vi "4155C QSCV Config SMUs v2.0.vi"(0 "VISA resource name in":refnum<visa-resource-name>, 1 "QSCV - Probe 4":u32(ring)=3 items=["SMU1  ", "SMU2  ", "SMU3  ", "SMU4  ", "SMU5  ", "SMU6  "], 2 "Gate mode":u16(ring) items=["Auto", "Limited", "Fixed"], 3 "Gate Range":u8(slide)=6 max=11 scale=0.0..11.0, 5 "QSCV - Source/Common":u32(ring) items=["SMU1  ", "SMU2  ", "SMU3  ", "SMU4  ", "SMU5  ", "SMU6  "], 7 "QSCV - Drain":u32(ring)=1 items=["SMU1  ", "SMU2  ", "SMU3  ", "SMU4  ", "SMU5  ", "SMU6  "], 9 "QSCV - Gate":u32(ring)=2 items=["SMU1  ", "SMU2  ", "SMU3  ", "SMU4  ", "SMU5  ", "SMU6  "], 11 "error in (no error)":errorcluster, 13 "Source/drain mode":u16(ring) items=["Auto", "Limited", "Fixed"], 14 "Source/drain Range":u8(slide)=6 max=11 scale=0.0..11.0) -> (4 "VISA Resource Name out":refnum<visa-resource-name>, 15 "error out":errorcluster)   [LabVIEW 2016]
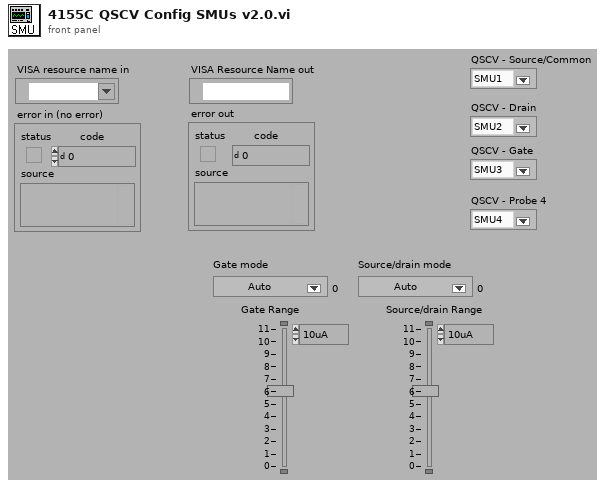
[diagram p1: front panel]
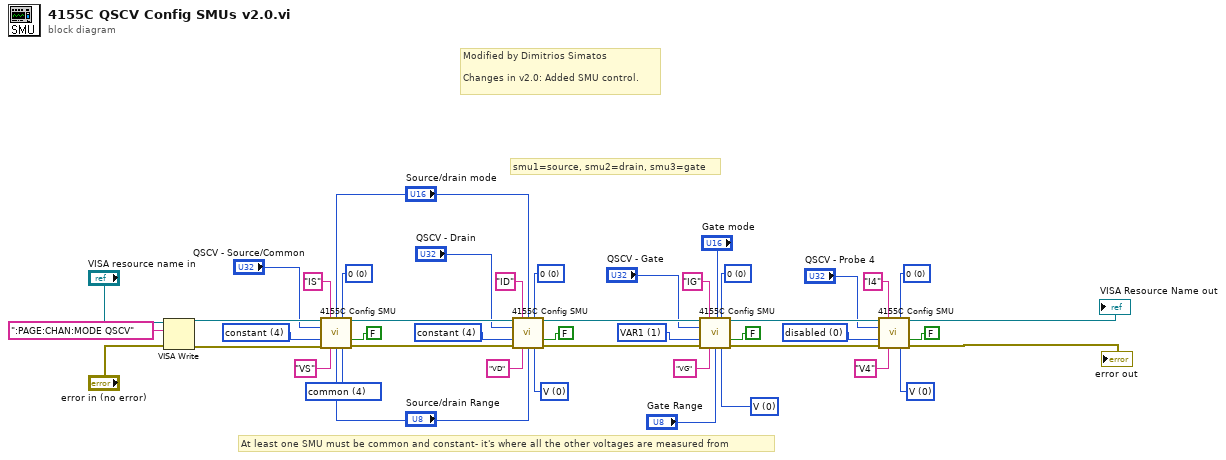
[diagram p0: block diagram]
diagram:
  w12 = u32 0 items=["V  ", "I  ", "V pulse  ", "I pulse  ", "  common  "] ("mode")
  w25 = u32 0 items=["V  ", "I  ", "V pulse  ", "I pulse  ", "  common  "] ("mode")
  w26 = u32 0 items=["0  ", "10K Ohms  ", "100K Ohms  ", "1M Ohms  "] ("series resistance *")
  w28 = u32 0 items=["disabled  ", "VAR1  ", "VAR2  ", "VAR1'  ", "constant  "] ("function")
  w31 = u32 0 items=["0  ", "10K Ohms  ", "100K Ohms  ", "1M Ohms  "] ("series resistance *")
  w33 = u32 1 items=["disabled  ", "VAR1  ", "VAR2  ", "VAR1'  ", "constant  "] ("function")
  w36 = u32 0 items=["V  ", "I  ", "V pulse  ", "I pulse  ", "  common  "] ("mode")
  w37 = u32 0 items=["0  ", "10K Ohms  ", "100K Ohms  ", "1M Ohms  "] ("series resistance *")
  w39 = u32 4 items=["disabled  ", "VAR1  ", "VAR2  ", "VAR1'  ", "constant  "] ("function")
  w42 = u32 4 items=["V  ", "I  ", "V pulse  ", "I pulse  ", "  common  "] ("mode")
  w43 = u32 0 items=["0  ", "10K Ohms  ", "100K Ohms  ", "1M Ohms  "] ("series resistance *")
  w45 = u32 4 items=["disabled  ", "VAR1  ", "VAR2  ", "VAR1'  ", "constant  "] ("function")
  # "Modified by Dimitrios Simatos\n\nChanges in v2.0: Added SMU control."
  # "smu1=source, smu2=drain, smu3=gate"
  # "At least one SMU must be common and constant- it's where all the other voltages are measured from"
  n1 = VISA Write(VISA resource name="VISA resource name in", write buffer=":PAGE:CHAN:MODE QSCV" ("write buffer (\"\")"), error in (no error)="error in (no error)") -> (VISA resource name out=w10:refnum<visa-resource-name>, error out=w11:errorcluster)  [unwired: 1 out]
  n2 = call "4155C Config SMU.vi"("VISA session"=w10, "I name (max 6 chars)"="IS", "Range mode"="Source/drain mode", "series resistance *"=w43, "unit to configure"="QSCV - Source/Common", "function"=w45, "standby"=FALSE, "error in (no error)"=w11, "V name (max 6 chars)"="VS", "Range"="Source/drain Range", "mode"=w42) -> ("dup VISA resource name"=w22:refnum<visa-resource-name>, "error out"=w21:errorcluster)  [unwired: 3 in]
  n3 = call "4155C Config SMU.vi"("VISA session"=w22, "I name (max 6 chars)"="ID", "Range mode"="Source/drain mode", "series resistance *"=w37, "unit to configure"="QSCV - Drain", "function"=w39, "standby"=FALSE, "error in (no error)"=w21, "V name (max 6 chars)"="VD", "Range"="Source/drain Range", "mode"=w36) -> ("dup VISA resource name"=w19:refnum<visa-resource-name>, "error out"=w20:errorcluster)  [unwired: 3 in]
  n4 = call "4155C Config SMU.vi"("VISA session"=w19, "I name (max 6 chars)"="IG", "Range mode"="Gate mode", "series resistance *"=w31, "unit to configure"="QSCV - Gate", "function"=w33, "standby"=FALSE, "error in (no error)"=w20, "V name (max 6 chars)"="VG", "Range"="Gate Range", "mode"=w12) -> ("dup VISA resource name"=w18:refnum<visa-resource-name>, "error out"=w17:errorcluster)  [unwired: 3 in]
  n5 = call "4155C Config SMU.vi"("VISA session"=w18, "I name (max 6 chars)"="I4", "series resistance *"=w26, "unit to configure"="QSCV - Probe 4", "function"=w28, "standby"=FALSE, "error in (no error)"=w17, "V name (max 6 chars)"="V4", "mode"=w25) -> ("dup VISA resource name"=→"VISA Resource Name out":refnum<visa-resource-name>, "error out"=→"error out":errorcluster)  [unwired: 5 in]
